vi "Close Child.vi"(8 "error in (no error)":errorcluster, 11 "VISA Client in":refnum<class "Serial Client.lvclass">) -> (0 "error out":errorcluster, 3 "VISA Client out":refnum<class "Serial Client.lvclass">)   [LabVIEW 2020, in "Stream-Serial.lvlib" / "Serial Client.lvclass"]
uses:
  Serial Client.lvclass
  Client Command.ctl
  Stream-Serial.lvlib
  lv-stream/stream/Connection/Connection.lvclass
  lv-stream/stream/Connection/State.ctl
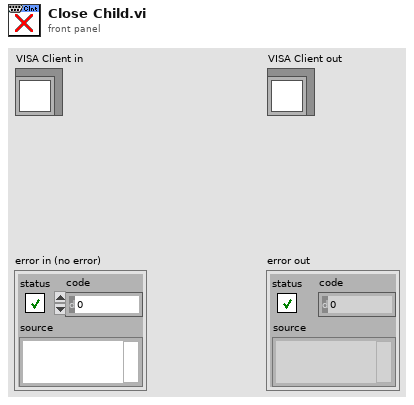
[diagram p1: front panel]
types:
  T1 = typedef "Stream.lvlib/Connection.lvclass/State.ctl" = enum16{"Closed", "Idle", "Connecting", "Connected", "Shutdown"}
  T2 = typedef "Stream-Serial.lvlib/Client Command.ctl" = enum16{"Connect", "Close", "Shutdown", "Reconnect"}
  T3 = typedef "Stream-Serial.lvlib/Command Queue.ctl" = refnum<queue>
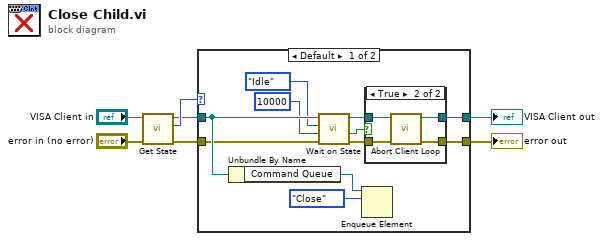
[diagram p0: block diagram]
diagram:
  n1 = call "Get State.vi"("error in (no error)"="error in (no error)", "Connection in"="VISA Client in") -> ("error out"=w1:errorcluster, "State"=w3:T1, "Connection out"=w2:refnum<class "Serial Client.lvclass">)  [unwired: 7 in]
  n2 = case shown="Default" w3 {
    tunnel: w2 -> [w14 w26]
    tunnel: w1 -> [w13 w25]
    tunnel: [w16 w26] -> w7
    tunnel: [w15 w25] -> w6
    frame Default {
      n3 = Unbundle By Name(w14) -> ("Command Queue"=w18:T3)
      n4 = call "Wait on State.vi"("error in (no error)"=w13, "Timeout ms (-1)"=10000, "State"=State."Idle", "Connection in"=w14) -> ("error out"=w9:errorcluster, "Timed Out?"=w8:bool, "Connection out"=w10:refnum<class "Serial Client.lvclass">)  [unwired: 5 in]
      n5 = Enqueue Element(queue=w18, element=Client_Command."Close") -> ()  [unwired: 2 in, 3 out]
      n6 = case shown="True" w8 {
        tunnel: w10 -> [w19 w23]
        tunnel: w9 -> [w20 w24]
        tunnel: [w19 w22] -> w16
        tunnel: [w20 w21] -> w15
        frame False {
        }
        frame True {
          n7 = call "Abort Client Loop.vi"("error in (no error)"=w24, "VISA Client in"=w23) -> ("error out"=w21:errorcluster, "VISA Client out"=w22:refnum<class "Serial Client.lvclass">)  [unwired: 8 in]
        }
      }
    }
    frame "Closed", "Idle" {
    }
  }
  "error out" <- w6
  "VISA Client out" <- w7
